vi "bytefiletweak.vi"() -> ()   [LabVIEW 2022 SP3]
panel:
  in  "Replace Skin?":bool
  in  "Rescale?":bool
  in  "Enum":enum16{"median", "3-D thresh", "add lines"}(ring)
  in  "lower threshold":i32=2
  in  "file extension to read":string="mbs"
  in  "threshold":i32=2
  in  "Save?":bool
  out "post Dimensions":i32[](array[numeric])
  out "after":u8[][](graph)
  in  "plane to view":i32
  out "before":u8[][](graph)
  in  "y pts":i32
  in  "x pts":i32
  in  "Choose Directory of Files":path=path "C:/WINDOWS/DESKTOP/rri.eye"
  out "pre Dimensions":i32[](array[numeric])
  in  "Number of planes":i32
  in  "Root name of file":string="plane"
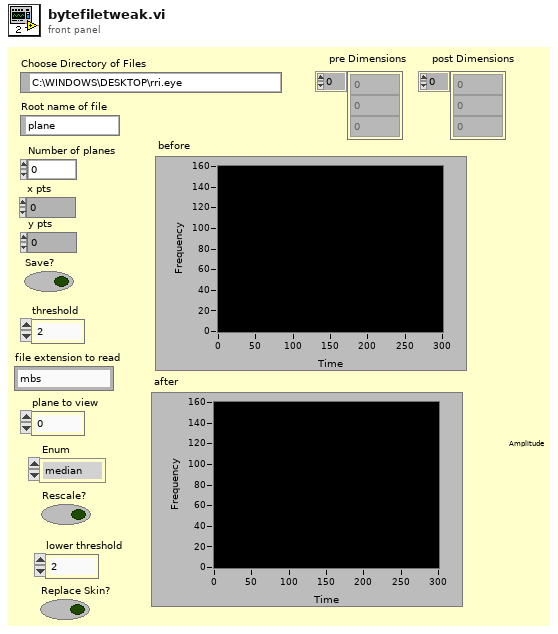
[diagram p1: front panel]
types:
  T1 = enum32{"existing file", "new file", "new or existing file", "existing dir", "new dir", "new or existing dir", "existing file (use LLBs)", "new file (use LLBs)", "new or existing file (use LLBs)", "new or existing file or directory (use LLBs)"}
  T2 = enum16{"open", "open or create", "create or replace", "create"}
  T3 = enum16{"open", "replace", "create", "open or create", "replace or create", "replace or create with confirmation"}
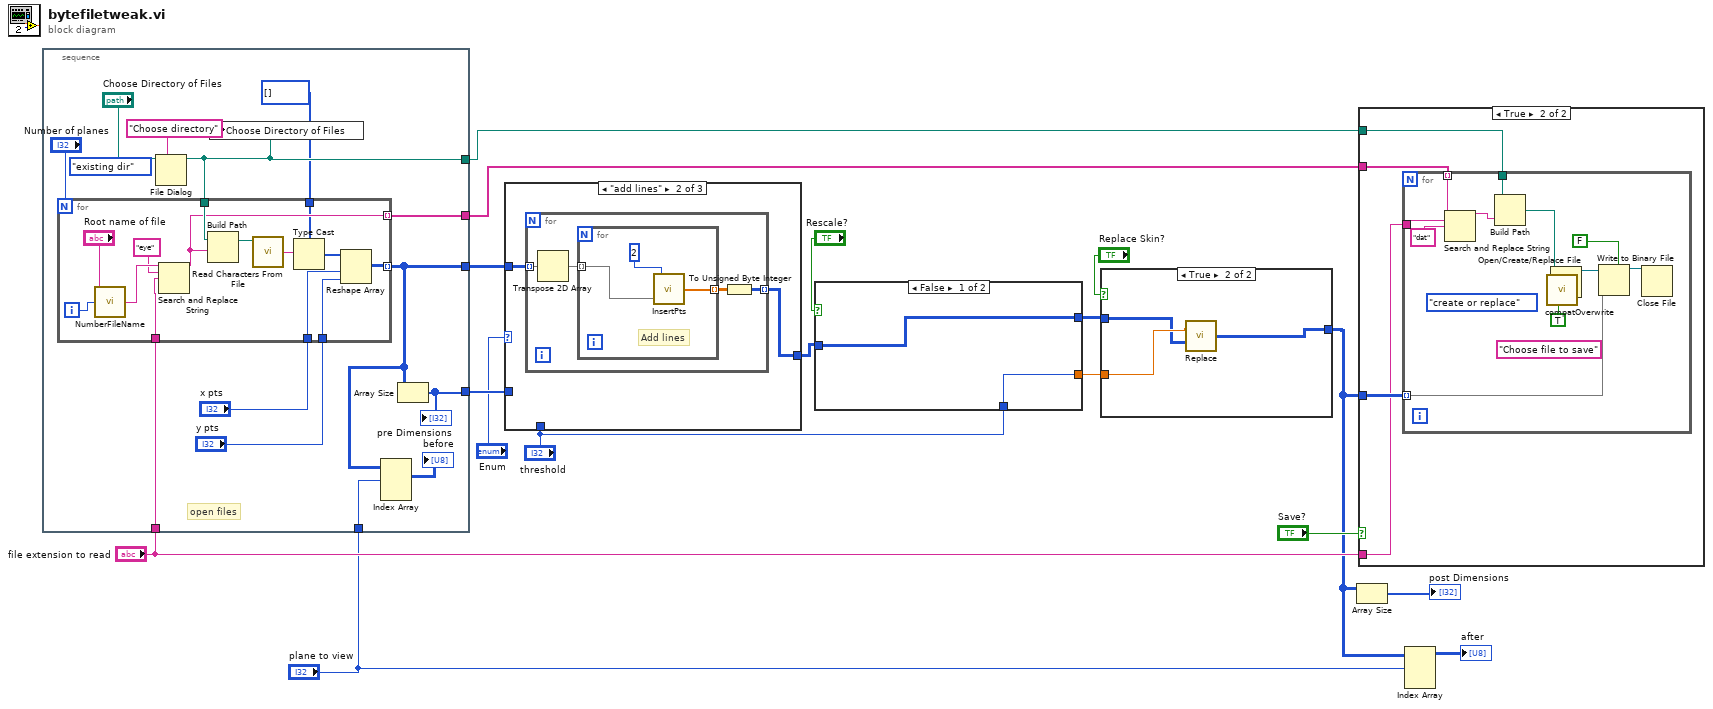
[diagram p0: block diagram]
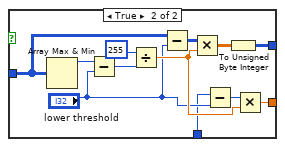
[diagram p3: hidden frame]
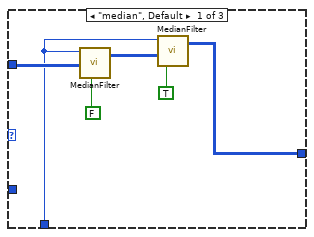
[diagram p4: hidden frame]
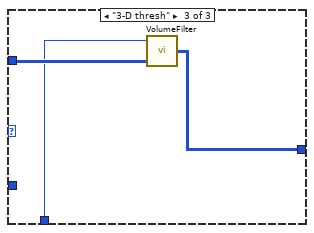
[diagram p5: hidden frame]
diagram:
  n1 = stacked-sequence {
    tunnel: [w20] -> w15
    tunnel: [w30] -> w17
    tunnel: [w29] -> w16
    tunnel: [w22] -> w14
    tunnel: "file extension to read" -> [w21]
    tunnel: "plane to view" -> [w19]
    frame #0 {
      (unwired) T1."existing dir" ("select mode (2)")
      # "open files"
      n2 = File Dialog(7:"Choose directory" ("prompt"), 11:"Choose Directory of Files") -> (3:w30:path)  [unwired: 5 in, 3 out]
      n3 = for {
        N: "Number of planes" -> [_]
        tunnel: w30 -> [w44]
        tunnel: [w32] -> w20 mode=indexing
        tunnel: u8[] [] ("Array Constant") -> [w34]
        tunnel: "x pts" -> [w39]
        tunnel: "y pts" -> [w38]
        tunnel: [w37] -> w29 mode=indexing
        tunnel: w21 -> [w31]
        i -> [w40]
        n4 = call "NumberFileName.vi"("File number"=w40, "file name"="Root name of file") -> ("Numbered File"=w42:string)  [unwired: 1 in]
        n5 = Search and Replace String(input string=w42, search string="eye", replace string=w31) -> (result string=w37:string)  [unwired: 5 in, 3 out]
        n6 = Build Path(base path=w44, name or relative path=w37) -> (appended path=w36:path)
        n7 = call <vilib>:"Read Characters From File.vi"("file path (dialog if empty)"=w36) -> ("character string"=w35:string)  [unwired: 5 in, 3 out]
        n8 = Type Cast(type=w34, x=w35) -> (*(type *) &x=w33:u8[])
        n9 = Reshape Array(w33, w39, w38) -> (w32:u8[][])
      }
      n10 = local write "Choose Directory of Files"(w30) -> ()
      n11 = Index Array(array=w20, index (dim 0)=w19) -> (element=→"before":u8[][])  [unwired: 2 in]
      n12 = Array Size(array=w20) -> (size(s)=w22:i32[])
      "pre Dimensions" <- w22
    }
  }
  n13 = case shown="\"add lines\"" "Enum" {
    tunnel: [w47 w51 w60] -> w5
    tunnel: w15 -> [w50 w52 w62]
    tunnel: w14 -> [_ _ _]
    tunnel: "threshold" -> [w48 _ w61]
    frame "median", Default {
      n14 = call "MedianFilter.vi"("Reverse"=FALSE, "data in"=w50, "threshold"=w48) -> ("data out"=w49:u8[][][])  [unwired: 4 in]
      n15 = call "MedianFilter.vi"("Reverse"=TRUE, "data in"=w49, "threshold"=w48) -> ("data out"=w47:u8[][][])  [unwired: 4 in]
    }
    frame "add lines" {
      n16 = for {
        tunnel: w52 -> [w56] mode=indexing
        tunnel: [w53] -> w51 mode=indexing
        n17 = Transpose 2D Array(2D array=w56) -> (transposed array=w54:u8[][])
        n18 = for {
          tunnel: w54 -> [w59] mode=indexing
          tunnel: [w57] -> w55 mode=indexing
          # "Add lines"
          n19 = call "InsertPts.vi"("Array in"=w59, "pts to insert"=2) -> ("Array ouput"=w57:dbl[])
        }
        n20 = To Unsigned Byte Integer(number=w55) -> (unsigned 8bit integer=w53:u8[][])
      }
      n21 = Array Size(array=w52) -> ()  [unwired: 1 out]
    }
    frame "3-D thresh" {
      n22 = call "VolumeFilter.vi"("data in"=w62, "threshold"=w61) -> ("Data Out"=w60:u8[][][])  [unwired: 1 in]
    }
  }
  n23 = case shown="False" "Rescale?" {
    tunnel: [w64 w72] -> w4
    tunnel: w5 -> [w64 w71]
    tunnel: "threshold" -> [w63 w66]
    tunnel: [w63 w65] -> w1
    frame False {
    }
    frame True {
      n24 = Array Max & Min(array=w71) -> (max value=w76:u8)  [unwired: 3 out]
      n25 = Subtract(x=w76, y="lower threshold") -> (x-y=w75:i32)
      n26 = Divide(x=255, y=w75) -> (x/y=w68:dbl)
      n27 = Subtract(x=w71, y="lower threshold") -> (x-y=w74:i32[][][])
      n28 = Multiply(x=w74, y=w68) -> (x*y=w73:dbl[][][])
      n29 = Subtract(x=w66, y="lower threshold") -> (x-y=w70:i32)
      n30 = To Unsigned Byte Integer(number=w73) -> (unsigned 8bit integer=w72:u8[][][])
      n31 = Multiply(x=w70, y=w68) -> (x*y=w65:dbl)
    }
  }
  n32 = case shown="True" "Replace Skin?" {
    tunnel: w4 -> [w77 w79]
    tunnel: [w77 w78] -> w3
    tunnel: w1 -> [_ w80]
    frame False {
    }
    frame True {
      n33 = call "Replace.vi"("data in"=w79, "threshold"=w80) -> ("data out"=w78:u8[][][])
    }
  }
  n34 = Array Size(array=w3) -> (size(s)=→"post Dimensions":i32[])
  n35 = case shown="True" "Save?" {
    tunnel: w3 -> [_ w82]
    tunnel: w17 -> [_ w84]
    tunnel: w16 -> [_ w83]
    tunnel: "file extension to read" -> [_ w81]
    frame False {
    }
    frame True {
      n36 = for {
        tunnel: w82 -> [w91] mode=indexing
        tunnel: w84 -> [w94]
        tunnel: w83 -> [w93] mode=indexing
        tunnel: w81 -> [w90]
        (unwired) "Choose file to save" ("prompt")
        (unwired) T2."create or replace" ("function (open:0)")
        n37 = Search and Replace String(input string=w93, search string=w90, replace string="dat") -> (result string=w96:string)  [unwired: 5 in, 3 out]
        n38 = Build Path(base path=w94, name or relative path=w96) -> (appended path=w88:path)
        n39 = call <vilib>:"compatOverwrite.vi"("overwrite (F)"=TRUE) -> ("overwrite?"=w86:T3)
        n40 = Open/Create/Replace File(file path (use dialog)=w88, operation (0:open)=w86) -> (refnum out=w89:refnum<file>)  [unwired: 4 in, 2 out]
        n41 = Write to Binary File(file (use dialog)=w89, data=w91, 5:FALSE ("prepend array or string size? (T)")) -> (refnum out=w92:refnum<file>)  [unwired: 3 in, 2 out]
        n42 = Close File(refnum=w92) -> ()  [unwired: 1 in, 2 out]
      }
    }
  }
  n43 = Index Array(array=w3, index (dim 0)="plane to view") -> (element=→"after":u8[][])  [unwired: 2 in]
